vi "generate.vi"(8 "error in (no error)":errorcluster, 11 "TrajectoryMG100122AODFrameScan in":refnum<class "TrajectoryMG100122AODFrameScan.lvclass">) -> (0 "error out":errorcluster, 3 "TrajectoryMG100122AODFrameScan out":refnum<class "TrajectoryMG100122AODFrameScan.lvclass">)   [LabVIEW 2010]
uses:
  fpga_VIs/FPGAMG100125AOD/FPGAMG100125AOD/FPGAMG100125AOD.lvclass
  TrajectoryMG100122AODFrameScan.lvclass
  FPGAWrapper/GenericFPGAWrapper/GenericFPGAWrapper/GenericFPGAWrapper.lvclass
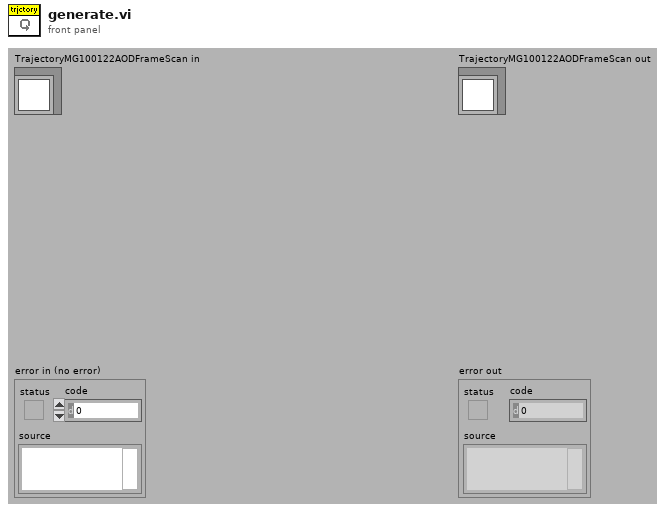
[diagram p1: front panel]
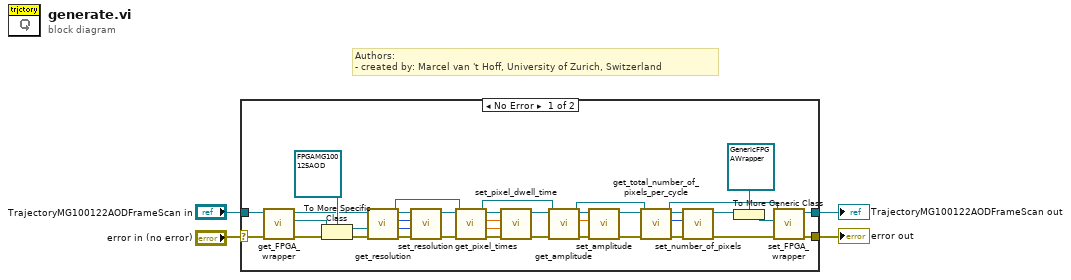
[diagram p0: block diagram]
diagram:
  # "Authors: \n- created by: Marcel van 't Hoff, University of Zurich, Switzerland"
  n1 = case shown="No Error" "error in (no error)" {
    selector: "error in (no error)" -> [w37 w40]
    tunnel: [w25 w40] -> w3
    tunnel: "TrajectoryMG100122AODFrameScan in" -> [w36 w39]
    tunnel: [w24 w39] -> w1
    frame No Error {
      n2 = call-dynamic "get_FPGA_wrapper.vi"("error in (no error)"=w37, "TrajectoryMG100122GenericFPGA in"=w36) -> ("error out"=w34:errorcluster, "GenericFPGAWrapper.lvclass"=w35:refnum<class "GenericFPGAWrapper.lvclass">, "TrajectoryMG100122GenericFPGA out"=w20:refnum<class "TrajectoryMG100122AODFrameScan.lvclass">)  [unwired: 7 in]
      n3 = To More Specific Class(target class=refnum<class "FPGAMG100125AOD.lvclass"> refnum ("FPGAMG100125AOD.lvclass"), reference=w35, error in=w34) -> (specific class reference=w18:refnum<class "FPGAMG100125AOD.lvclass">, error out=w21:errorcluster)
      n4 = call-dynamic "get_resolution.vi"("error in (no error)"=w21, "TrajectoryMG100122AODFrameScan in"=w20) -> ("error out"=w16:errorcluster, "y resolution"=w13:i32, "x resolution"=w14:i32, "TrajectoryMG100122AODFrameScan out"=w19:refnum<class "TrajectoryMG100122AODFrameScan.lvclass">)  [unwired: 6 in]
      n5 = call-dynamic "set_resolution.vi"("error in (no error)"=w16, "y"=w13, "x"=w14, "FPGAMG100125AOD in"=w18) -> ("error out"=w15:errorcluster, "FPGAMG100125AOD out"=w17:refnum<class "FPGAMG100125AOD.lvclass">)  [unwired: 6 in]
      n6 = call-dynamic "get_pixel_times.vi"("error in (no error)"=w15, "TrajectoryMG100122AODFrameScan in"=w19) -> ("error out"=w31:errorcluster, "AOD equilibration time"=w32:dbl[unit], "pixel dwell time"=w33:dbl[unit], "TrajectoryMG100122AODFrameScan out"=w29:refnum<class "TrajectoryMG100122AODFrameScan.lvclass">)  [unwired: 6 in]
      n7 = call-dynamic "set_pixel_dwell_time.vi"("error in (no error)"=w31, "AOD equilibration time"=w32, "pixel dwell time"=w33, "FPGAMG100125AOD in"=w17) -> ("error out"=w30:errorcluster, "FPGAMG100125AOD out"=w26:refnum<class "FPGAMG100125AOD.lvclass">)  [unwired: 6 in]
      n8 = call-dynamic "get_amplitude.vi"("error in (no error)"=w30, "TrajectoryMG100122AODFrameScan in"=w29) -> ("error out"=w28:errorcluster, "AOD amplitude"=w27:dbl, "TrajectoryMG100122AODFrameScan out"=w12:refnum<class "TrajectoryMG100122AODFrameScan.lvclass">)  [unwired: 7 in]
      n9 = call-dynamic "set_amplitude.vi"("error in (no error)"=w28, "AOD amplitude"=w27, "FPGAMG100125AOD in"=w26) -> ("error out"=w10:errorcluster, "FPGAMG100125AOD out"=w9:refnum<class "FPGAMG100125AOD.lvclass">)  [unwired: 7 in]
      n10 = call-dynamic "get_total_number_of_pixels_per_cycle.vi"("error in (no error)"=w10, "TrajectoryMG100122AODFrameScan in"=w12) -> ("error out"=w7:errorcluster, "total number of pixels per cycle"=w5:i32, "TrajectoryMG100122AODFrameScan out"=w11:refnum<class "TrajectoryMG100122AODFrameScan.lvclass">)  [unwired: 7 in]
      n11 = call-dynamic "set_number_of_pixels.vi"("error in (no error)"=w7, "number of pixels"=w5, "FPGAMG100125AOD in"=w9) -> ("error out"=w6:errorcluster, "FPGAMG100125AOD out"=w8:refnum<class "FPGAMG100125AOD.lvclass">)  [unwired: 7 in]
      n12 = To More Generic Class(target class=refnum<class "GenericFPGAWrapper.lvclass"> refnum ("GenericFPGAWrapper.lvclass"), reference=w8) -> (generic class reference=w22:refnum<class "GenericFPGAWrapper.lvclass">)
      n13 = call-dynamic "set_FPGA_wrapper.vi"("error in (no error)"=w6, "GenericFPGAWrapper.lvclass"=w22, "TrajectoryMG100122GenericFPGA in"=w11) -> ("error out"=w25:errorcluster, "TrajectoryMG100122GenericFPGA out"=w24:refnum<class "TrajectoryMG100122AODFrameScan.lvclass">)  [unwired: 7 in]
    }
    frame Error {
    }
  }
  "error out" <- w3
  "TrajectoryMG100122AODFrameScan out" <- w1
